vi "RSZVB Set Time Domain Time Span.vi"(8 "error in (no error)":errorcluster {"code" format="%.0x"}, 9 "Time Span (5.0E-9 s)":dbl=5e-09 format="%^.3e", 10 "Channel (Trace) (1)":i32=1, 11 "VISA session":refnum<visa-resource-name>) -> (0 "error out":errorcluster {"code" format="%.0x"}, 3 "dup VISA session":refnum<visa-resource-name>)   [LabVIEW 2011]
doc: "This VI defines the time span of the diagram in time domain.\n\nRemote-control command(s):\nCALCulate<Ch/Tr>:TRANsform:TIME:SPAN"
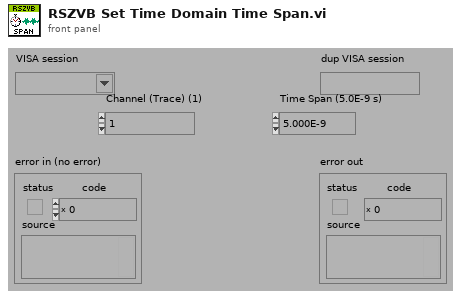
[diagram p1: front panel]
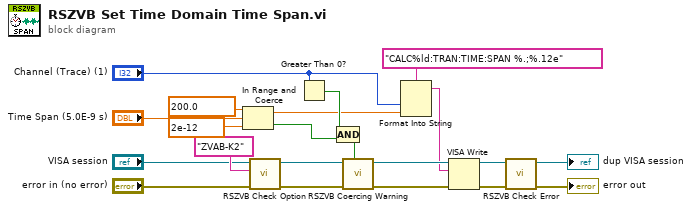
[diagram p0: block diagram]
diagram:
  n1 = In Range and Coerce(upper limit=200.0, x="Time Span (5.0E-9 s)", lower limit=2e-12) -> (coerced(x)=w8:dbl, In Range?=w9:bool)
  n2 = call "RSZVB Check Option.vi"("error in (no error)"="error in (no error)", "Options"="ZVAB-K2", "VISA session"="VISA session") -> ("error out"=w7:errorcluster, "dup VISA session"=w12:refnum<visa-resource-name>)  [unwired: 7 in]
  n3 = Greater Than 0?(x="Channel (Trace) (1)") -> (x > 0?=w14:bool)
  n4 = Compound Arithmetic op=AND(w14, w9) -> (w16:bool)
  n5 = call "RSZVB Coercing Warning.vi"("In Range?"=w16, "error in (no error)"=w7, "VISA session"=w12) -> ("error out"=w19:errorcluster, "dup VISA session"=w20:refnum<visa-resource-name>)  [unwired: 7 in]
  n6 = Format Into String(format string="CALC%ld:TRAN:TIME:SPAN %.;%.12e", "Channel (Trace) (1)", w8) -> (resulting string=w15:string)  [unwired: 2 in, 1 out]
  n7 = VISA Write(VISA resource name=w20, write buffer=w15, error in (no error)=w19) -> (VISA resource name out=w17:refnum<visa-resource-name>, error out=w18:errorcluster)  [unwired: 1 out]
  n8 = call "RSZVB Check Error.vi"("error in (no error)"=w18, "VISA session"=w17) -> ("error out"=→"error out":errorcluster, "dup VISA session"=→"dup VISA session":refnum<visa-resource-name>)  [unwired: 8 in]
